vi "CPC ESF Example.vi"() -> ()   [LabVIEW 2014, in "CPC.lvclass"]
uses:
  CPC.lvclass
  reusable/Session APIs/Serial/Serial Session.lvclass
  <userlib>/_Session Fwk/Session - Root.lvclass
  reusable/Session APIs/File Access/Config Data/Config Data.lvclass
  reusable/Session APIs/File Access/Config Data/Config Session.ctl
  Controls/3022A/Flow.ctl
panel:
  out "current time":timestamp
  in  "Flow Rate In":T1
  out "Tsaturator":dbl
  out "Tcondenser":dbl
  out "FP Concentration":dbl
  out "Buffer - 2s":u32
  out "Buffer - 1s":i32
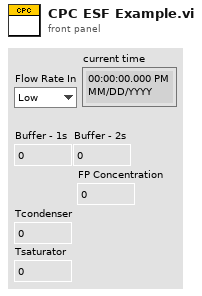
[diagram p1: front panel]
types:
  T1 = typedef "CPC.lvclass/Flow.ctl" = enum16{"Low", "High"}
  T2 = typedef "Config Data.lvclass/Config Session.ctl" = refnum<data-value>
  T3 = typedef "Session - Root.lvclass/Session Handle.ctl" = refnum<data-value>
  T4 = typedef "Serial Session.lvclass/Session Handle.ctl" = refnum<data-value>
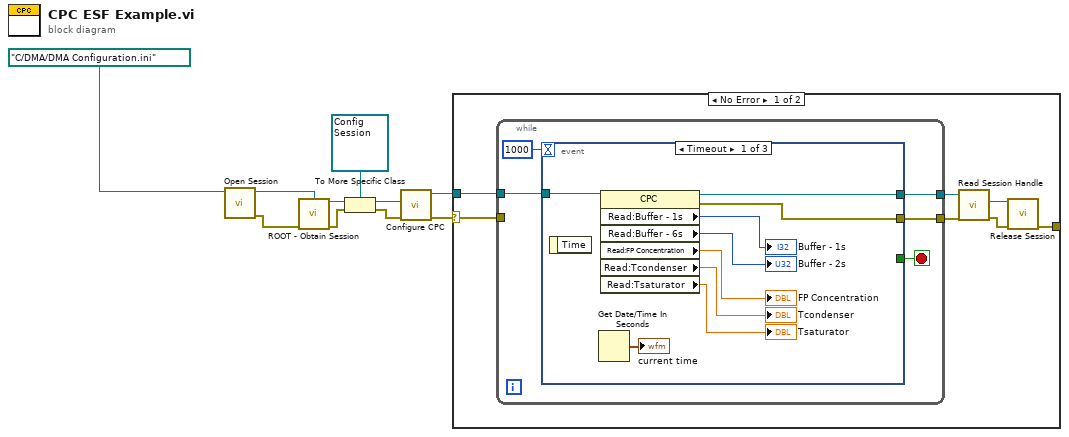
[diagram p0: block diagram]
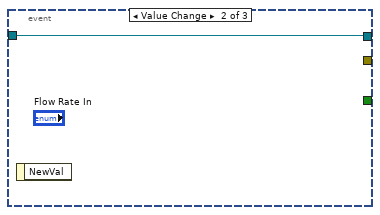
[diagram p2: hidden frame]
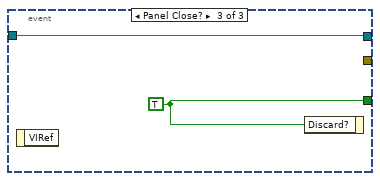
[diagram p3: hidden frame]
diagram:
  n1 = call "Open Session.vi"("Path"=path "C:/DMA/DMA Configuration.ini") -> ("error out"=w2:errorcluster, "Config Data"=w7:refnum<class "Config Data.lvclass">)  [unwired: 9 in]
  n2 = call <userlib>:"ROOT - Obtain Session.vi"("OBJ - Session"=w7, "error in (no error)"=w2) -> ("Session Handle"=w6:T3, "error out"=w1:errorcluster)  [unwired: 11 in, 1 out]
  n3 = To More Specific Class(target class=T2 refnum ("Session Handle"), reference=w6, error in=w1) -> (specific class reference=w4:T2, error out=w3:errorcluster)
  n4 = call "Configure CPC.vi"("error in"=w3, "Config Handle"=w4) -> ("error out"=w10:errorcluster, "CPC out"=w9:refnum<class "CPC.lvclass">)  [unwired: 8 in]
  n5 = case shown="No Error" w10 {
    selector: w10 -> [w13 _]
    tunnel: [w15 _] -> _
    tunnel: w9 -> [w14 _]
    frame No Error {
      n6 = while {
        tunnel: w13 -> [_]
        tunnel: w14 -> [w21]
        tunnel: [w20] -> w17
        tunnel: [w18] -> w12
        stop <- w19 stop-if-true
        n7 = event shown="[0] Timeout" {
          selector: _ -> [_ _ _]
          dyn-events: _ -> [_ _ _]
          timeout: 1000 -> [_ _ _]
          tunnel: w21 -> [w31 w32 w33]
          tunnel: [w30 w32 w33] -> w20
          tunnel: [w29 _ _] -> w18
          tunnel: [_ _ w34] -> w19
          event Timeout {
            n8 = event-data() -> ()  [unwired: 1 in, 1 out]
            n9 = Get Date/Time In Seconds() -> (seconds since 1Jan1904=→"current time":timestamp)
            n10 = property class="CPC"(reference=w31) -> (reference out=w30:refnum<class "CPC.lvclass">, error out=w29:errorcluster, "Read:Buffer - 1s"=→"Buffer - 1s":i32, "Read:Buffer - 6s"=→"Buffer - 2s":u32, "Read:FP Concentration"=→"FP Concentration":dbl, "Read:Tcondenser"=→"Tcondenser":dbl, "Read:Tsaturator"=→"Tsaturator":dbl)  [unwired: 1 in]
          }
          event Value Change {
            n11 = event-data() -> ()  [unwired: 1 in, 1 out]
          }
          event Panel Close? {
            w34 = TRUE
            n12 = event-data() -> ()  [unwired: 1 in, 1 out]
            n13 = event-data("Discard?"=w34) -> ()  [unwired: 1 in, 1 out]
          }
        }
      }
      n14 = call "Read Session Handle.vi"("error in (no error)"=w12, "CPC in"=w17) -> ("error out"=w11:errorcluster, "Session Handle"=w16:T4)  [unwired: 7 in, 1 out]
      n15 = call "Release Session.vi"("Session Handle"=w16, "error in (no error)"=w11) -> ("error out"=w15:errorcluster)  [unwired: 13 in]
    }
    frame Error {
    }
  }
